vi "_write.vi"(8 "Error in (no error)":errorcluster, 10 "Log in":T1 {"Priority" items=["EMERGENCY", "ALERT", "CRITICAL", "ERROR", "WARNING", "NOTICE", "INFO", "DEBUG"]}, 11 "LogWriterMock in":refnum<class "LogWriterMock.lvclass">) -> (0 "Error out":errorcluster, 3 "LogWriterMock out":refnum<class "LogWriterMock.lvclass">)   [LabVIEW 2011, in "LogWriterMock.lvclass"]
uses:
  LogWriterMock.lvclass
  Log/LogCluster.ctl
  Log/PrioritiesRing.ctl
  LogWriterMock.lvclass/LogWriterMock.ctl
  Log/Log.lvclass
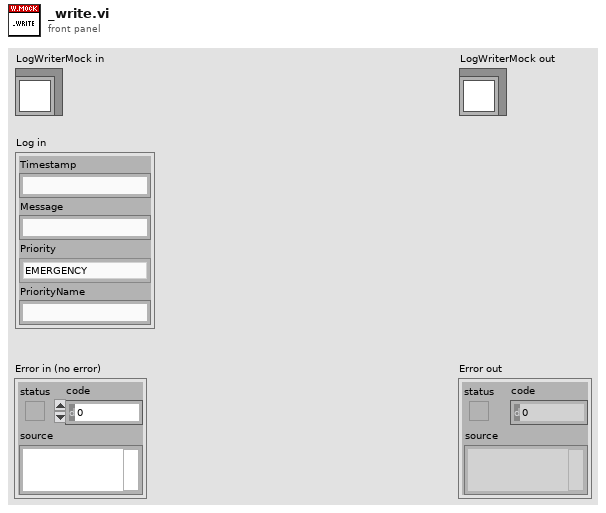
[diagram p1: front panel]
types:
  T1 = typedef "Log.lvclass/LogCluster.ctl" = cluster{"Timestamp":string, "Message":string, "Priority":T2, "PriorityName":string}
  T2 = typedef "Log.lvclass/PrioritiesRing.ctl" = u32
  T3 = typedef "Log.lvclass/Buffer.ctl" = u32
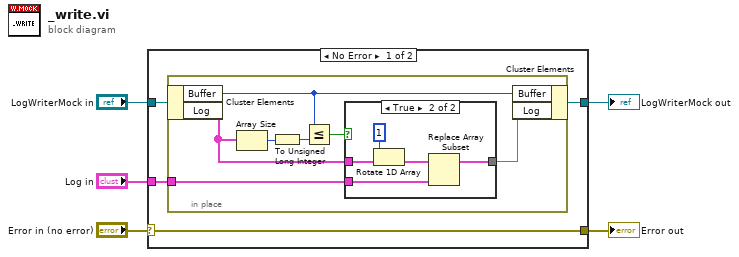
[diagram p0: block diagram]
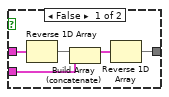
[diagram p2: hidden frame]
diagram:
  n1 = case shown="No Error" "Error in (no error)" {
    selector: "Error in (no error)" -> [w9 w28]
    tunnel: [w9 w28] -> w4
    tunnel: [w7 w27] -> w2
    tunnel: "LogWriterMock in" -> [w8 w27]
    tunnel: "Log in" -> [w6 _]
    frame No Error {
      n2 = in-place {
        in-place-border: w6 -> [w12]
        n3 = in-place-cluster #1(w8) -> ("Buffer"=w15:T3, "Log"=w11:T1[])
        n4 = Array Size(array=w11) -> (size(s)=w16:i32)
        n5 = To Unsigned Long Integer(number=w16) -> (unsigned 32bit integer=w14:u32)
        n6 = Less Or Equal?(x=w15, y=w14) -> (x <= y?=w13:bool)
        n7 = case shown="True" w13 {
          tunnel: w12 -> [w19 w23]
          tunnel: w11 -> [w21 w26]
          tunnel: [w17 w22] -> w10
          frame False {
            n8 = Reverse 1D Array(array=w21) -> (reversed array=w20:T1[])
            n9 = Build Array (concatenate)(w20, w19) -> (w18:T1[])
            n10 = Reverse 1D Array(array=w18) -> (reversed array=w17:T1[])
          }
          frame True {
            n11 = Rotate 1D Array(1:w26, 2:1 ("n")) -> (0:w24:T1[])
            n12 = Replace Array Subset(array=w24, new element=w23) -> (w22:T1[])  [unwired: 1 in]
          }
        }
        n13 = in-place-cluster #1("Buffer"=w15, "Log"=w10) -> (w7:refnum<class "LogWriterMock.lvclass">)
      }
    }
    frame Error {
    }
  }
  "Error out" <- w4
  "LogWriterMock out" <- w2
